vi "Stream Basic with Config.vi"() -> ()   [LabVIEW 2020]
panel:
  out "Combined DIO17 Count":i32
  out "Combined DIO16 Count":i32
  in  "Config Values":dbl[](array[numeric])=[10.0, 0.0, 0.0, 0.0, 0.0, 0.0, 0.0, 0.0, 7.0, 1.0, 0.0, 7.0, 1.0] format="%.2f"
  in  "Config Names":string[](array[string])=["AIN_ALL_RANGE", "STREAM_SETTLING_US", "STREAM_RESOLUTION_INDEX", "STREAM_BUFFER_SIZE_BYTES", "DIO_EF_CLOCK0_ENABLE", "DIO_EF_CLOCK1_ENABLE", "DIO_EF_CLOCK2_ENABLE", "DIO16_EF_ENABLE", "DIO16_EF_INDEX", "DIO16_EF_ENABLE", "DIO17_EF_ENABLE", "DIO17_EF_INDEX", "DIO17_EF_ENABLE"]
  in  "#Seconds on Graph":dbl=1.0 format="%.2f"
  out "ScansPerRead":i32=500
  out "ConnectionType Out":i32=1
  out "DeviceType Out":i32=7
  in  "Identifier":string="LJM_idANY"
  in  "ConnectionType":string="LJM_ctANY"
  in  "DeviceType":string="LJM_dtANY"
  out "DeviceScanBacklog":i32
  out "LJMScanBacklog":i32
  out "Data":dbl[][](array[numeric]) format="%.3f"
  out "Waveform Graph":dbl[][](graph)
  in  "Scan List":string[](array[string])=["AIN0", "DIO16_EF_READ_A", "STREAM_DATA_CAPTURE_16", "DIO17_EF_READ_A", "STREAM_DATA_CAPTURE_16"]
  out "# of iterations":i32
  in  "Scan Rate (Hz)":dbl=1000.0 format="%.3f"
  in  "stop":bool
  out "Error Message":string
  # "To remove an element, right-click\non it, select Data Operations =>\nRemove Element.\n\nTo empty an array, right-click\nnear the edge, select Data\nOperations => Empty Array.\n\nOther useful operations:  From the\nOperate menu are \"Make Current\nValues Default\" and \"Reinitialize\nTo Default\"."
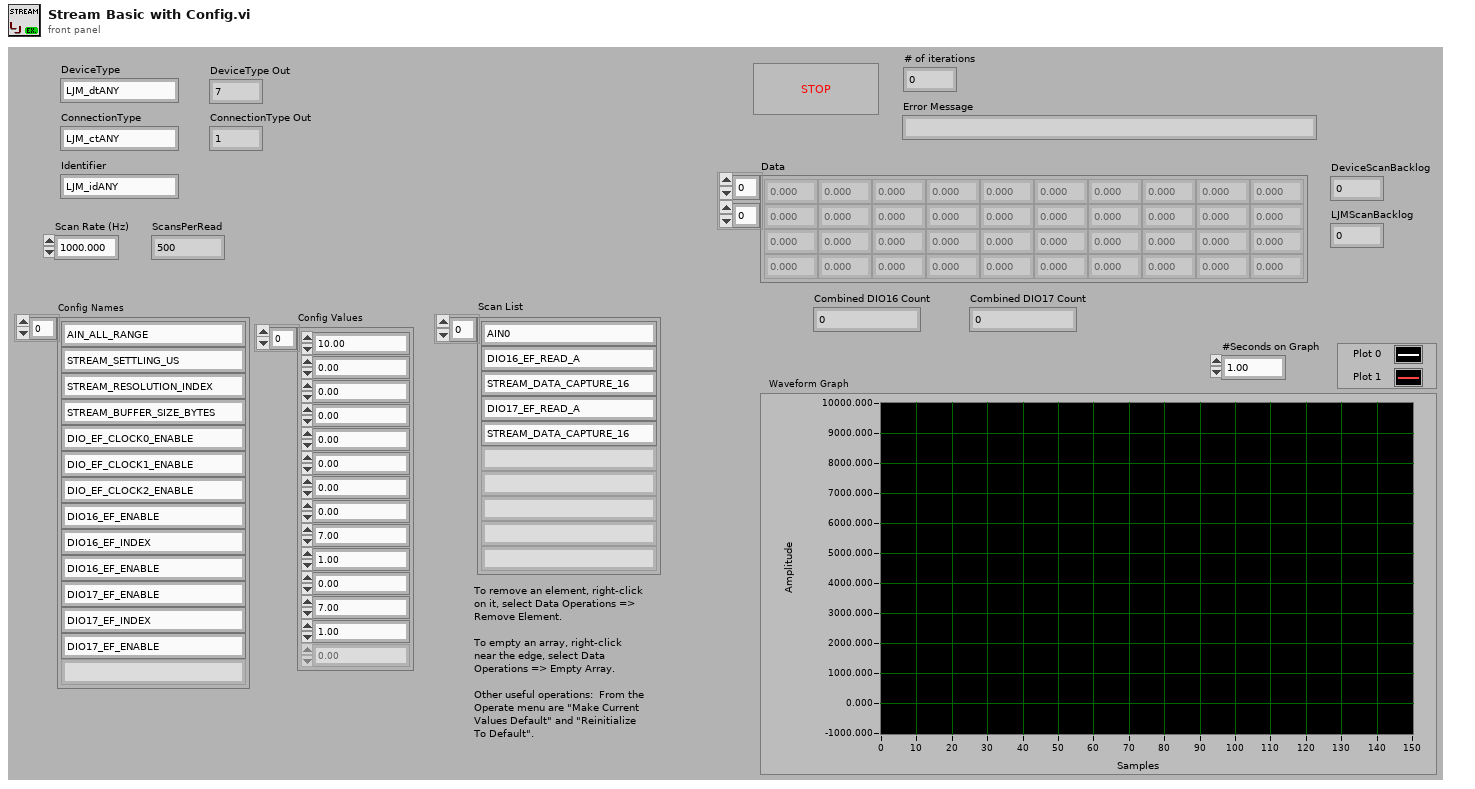
[diagram p1: front panel]
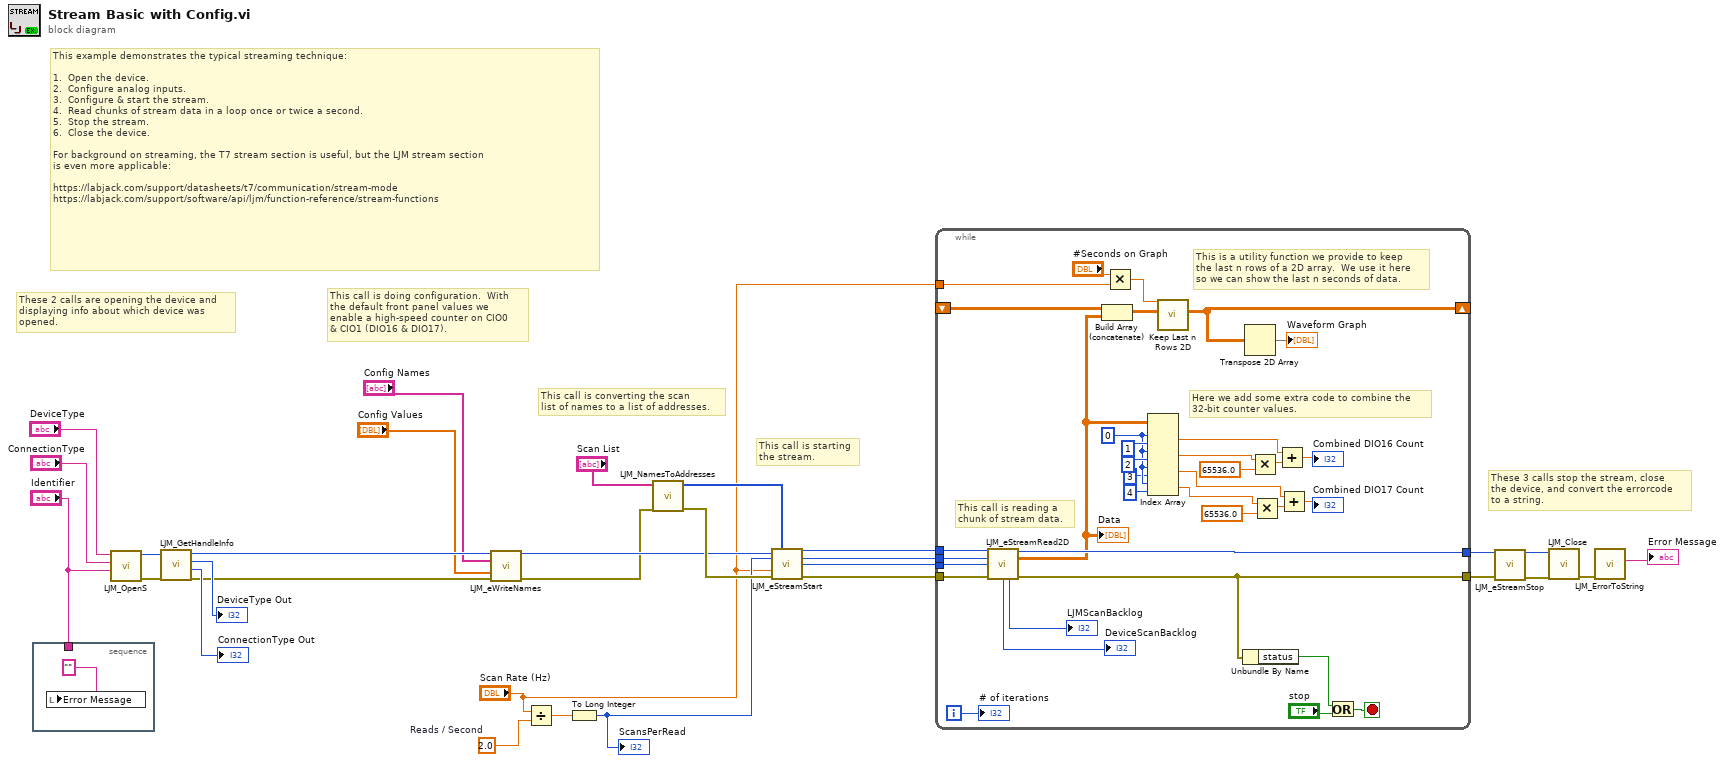
[diagram p0: block diagram]
diagram:
  w14 = 2.0  # Reads / Second
  # "This example demonstrates the typical streaming technique:\n\n1.  Open the device.\n2.  Configure analog inputs.\n3.  Configure & start the stream.\n4.  Read chunks of stream data in a loop once or twice a second.\n5.  Stop the stream.\n6.  Close the device.\n\nFor background on streaming, the T7 stream section is useful, but the LJM stream section\nis even more applicable:\n\nhttps://labjack.com/support/datasheets/t7/communication/stream-mode\nhttps://labjack.com/support/software/api/ljm/function-reference/stream-functions"
  # "These 3 calls stop the stream, close\nthe device, and convert the errorcode\nto a string."
  # "This call is starting\nthe stream."
  # "This call is converting the scan\nlist of names to a list of addresses."
  # "This call is doing configuration.  With\nthe default front panel values we\nenable a high-speed counter on CIO0\n& CIO1 (DIO16 & DIO17)."
  # "These 2 calls are opening the device and\ndisplaying info about which device was\nopened."
  n1 = stacked-sequence {
    tunnel: "Identifier" -> [_]
    frame #0 {
      n2 = local write "Error Message"("" ("Error Message")) -> ()
    }
  }
  n3 = call "LJM_OpenS.vi"("Identifier"="Identifier", "ConnectionType"="ConnectionType", "DeviceType"="DeviceType") -> ("error out"=w22:errorcluster, "Handle"=w19:i32)  [unwired: 7 in]
  n4 = call "LJM_GetHandleInfo.vi"("error in"=w22, "Handle In"=w19) -> ("error out"=w11:errorcluster, "ConnectionType"=→"ConnectionType Out":i32, "DeviceType"=→"DeviceType Out":i32, "Handle Out"=w10:i32)  [unwired: 2 in, 4 out]
  n5 = call "LJM_eWriteNames.vi"("Handle In"=w10, "aNames"="Config Names", "aValuesIn"="Config Values", "error in"=w11) -> ("Handle Out"=w9:i32, "error out"=w8:errorcluster)  [unwired: 9 in, 1 out]
  n6 = Divide(x="Scan Rate (Hz)", y=w14) -> (x/y=w13:dbl)
  n7 = To Long Integer(number=w13) -> (32bit integer=w12:i32)
  "ScansPerRead" <- w12
  n8 = call "LJM_NamesToAddresses.vi"("error in"=w8, "aNames"="Scan List") -> ("error out"=w15:errorcluster, "aAddresses"=w7:i32[])  [unwired: 7 in, 1 out]
  n9 = call "LJM_eStreamStart.vi"("Handle In"=w9, "aScanList"=w7, "ScansPerRead"=w12, "ScanRate"="Scan Rate (Hz)", "error in"=w15) -> ("Handle Out"=w29:i32, "ScansPerRead Out"=w4:i32, "NumReadAddresses"=w5:i32, "error out"=w30:errorcluster)  [unwired: 5 in, 2 out]
  n10 = while {
    tunnel: [w60] -> w27
    tunnel: w29 -> [w61]
    tunnel: w5 -> [w56]
    tunnel: w4 -> [w55]
    shift-right: [w48] -> _
    shift-left: _ -> [w52]
    tunnel: "Scan Rate (Hz)" -> [w51]
    tunnel: w30 -> [w62]
    tunnel: [w57] -> w28
    i -> [w63]
    stop <- w64 stop-if-true
    w40 = 0 ("index (row)")
    # "Here we add some extra code to combine the\n32-bit counter values."
    # "This call is reading a\nchunk of stream data."
    # "This is a utility function we provide to keep\nthe last n rows of a 2D array.  We use it here\nso we can show the last n seconds of data."
    n11 = call "LJM_eStreamRead2D.vi"("Handle In"=w61, "ScansPerRead"=w55, "NumAddresses"=w56, "error in"=w62) -> ("Handle Out"=w60:i32, "aData Out"=w47:dbl[][], "DeviceScanBacklog"=→"DeviceScanBacklog":i32, "LJMScanBacklog"=→"LJMScanBacklog":i32, "error out"=w57:errorcluster)  [unwired: 7 in]
    "Data" <- w47
    n12 = Build Array (concatenate)(w52, w47) -> (w50:dbl[][])
    n13 = Multiply(x="#Seconds on Graph", y=w51) -> (x*y=w49:dbl)
    n14 = Index Array(array=w47, index (row) #1=w40, index (col) #1=1 ("disabled index (col)"), index (row) #2=w40, index (col) #2=2 ("disabled index (col)"), index (row) #3=w40, index (col) #3=3 ("disabled index (col)"), index (row) #4=w40, index (col) #4=4 ("disabled index (col)")) -> (element #1=w37:dbl, element #2=w36:dbl, element #3=w35:dbl, element #4=w34:dbl)
    n15 = call "Keep Last n Rows 2D.vi"("Array"=w50, "# Rows to Keep"=w49) -> ("Last n Rows"=w48:dbl[][])  [unwired: 9 in]
    n16 = Unbundle By Name(w57) -> ("status"=w65:bool)
    n17 = Transpose 2D Array(2D array=w48) -> (transposed array=→"Waveform Graph":dbl[][])
    n18 = Multiply(x=w36, y=65536.0) -> (x*y=w46:dbl)
    n19 = Multiply(x=w34, y=65536.0) -> (x*y=w43:dbl)
    n20 = Add(x=w37, y=w46) -> (x+y=→"Combined DIO16 Count":dbl)
    n21 = Add(x=w35, y=w43) -> (x+y=→"Combined DIO17 Count":dbl)
    n22 = Or(x=w65, y="stop") -> (x .or. y?=w64:bool)
    "# of iterations" <- w63
  }
  n23 = call "LJM_eStreamStop.vi"("Handle In"=w27, "error in"=w28) -> ("Handle Out"=w25:i32, "error out"=w26:errorcluster)  [unwired: 12 in]
  n24 = call "LJM_Close.vi"("error in"=w26, "Handle"=w25) -> ("error out"=w24:errorcluster)  [unwired: 9 in]
  n25 = call "LJM_ErrorToString.vi"("error in"=w24) -> ("String"=→"Error Message":string)  [unwired: 10 in]
